vi "SerializeBuildHeader.vi"(8 "error in (no error)":errorcluster, 10 "PlaceholderData?":bool[](array[boolean]), 11 "All class layers":T1[](array[typedef])) -> (0 "error out":errorcluster, 2 "Version header":variant, 3 "Class header":variant)   [LabVIEW 2020, in "BlueSerialization.lvlib" / "BlueSerializer.lvclass"]
uses:
  BlueSerializer.lvclass
  Support/GetSerializableDataClusterClass.ctl
  Support/SerializableDataGetDataAction.ctl
  ClassNameAndVersion.ctl
  <vilib>/Utility/EditLVLibs/LibVersion.ctl
  <vilib>/Utility/error.llb/Error Cluster From Error Code.vi
  <vilib>/ErrorRing/Error Ring.xnode
  <vilib>/Utility/EditLVLibs/Edit LVLibs.lvlib
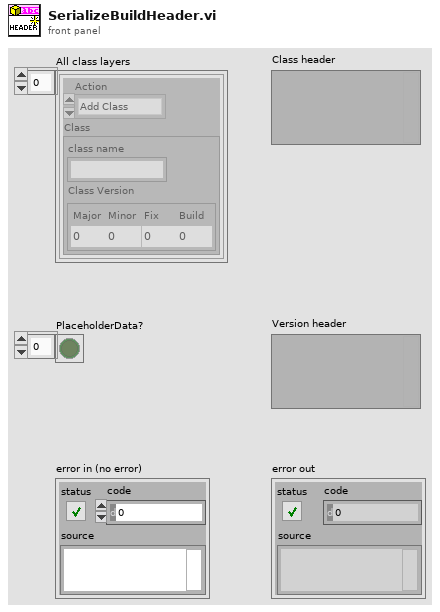
[diagram p1: front panel]
types:
  T1 = typedef "BlueSerialization.lvlib/BlueSerializer.lvclass/GetSerializableDataClusterClass.ctl" = cluster{"Action":T2, "Class":T3}
  T2 = typedef "BlueSerialization.lvlib/BlueSerializer.lvclass/SerializableDataGetDataAction.ctl" = enum16{"Add Class", "Drop Class"}
  T3 = typedef "BlueSerialization.lvlib/BlueSerializer.lvclass/ClassNameAndVersion.ctl" = cluster{"class name":string, "Class Version":T4}
  T4 = typedef "Edit LVLibs.lvlib/LibVersion.ctl" = cluster{"Major":u16, "Minor":u16, "Fix":u16, "Build":u16}
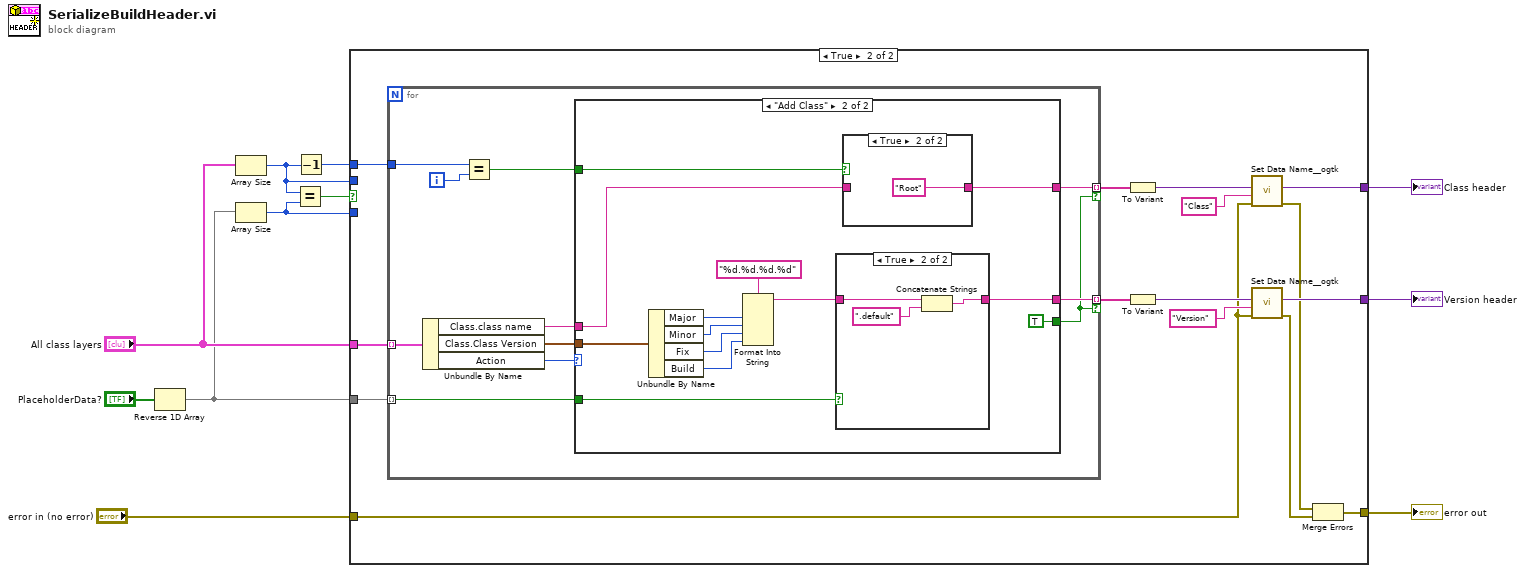
[diagram p0: block diagram]
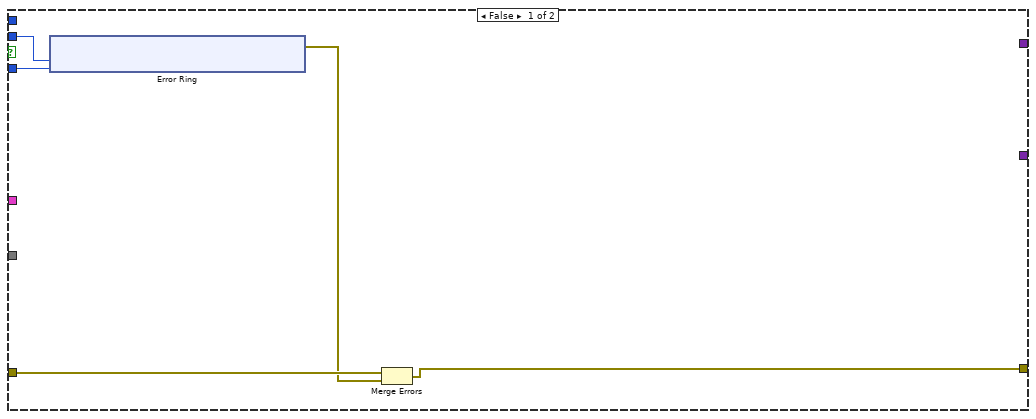
[diagram p2: hidden frame]
diagram:
  n1 = Reverse 1D Array(array="PlaceholderData?") -> (reversed array=w1:bool[])
  n2 = Array Size(array="All class layers") -> (size(s)=w3:i32)
  n3 = Array Size(array=w1) -> (size(s)=w4:i32)
  n4 = Equal?(x=w3, y=w4) -> (x = y?=w5:bool)
  n5 = Decrement(x=w3) -> (x-1=w8:i32)
  n6 = case shown="True" w5 {
    tunnel: [_ w34] -> w11
    tunnel: [_ w33] -> w10
    tunnel: "All class layers" -> [_ w32]
    tunnel: w8 -> [_ w30]
    tunnel: "error in (no error)" -> [w14 w29]
    tunnel: [w12 w27] -> w6
    tunnel: w1 -> [_ w25]
    tunnel: w4 -> [w16 _]
    tunnel: w3 -> [w15 _]
    frame False {
      n7 = xnode "Error Ring"("parameter 0"=w15, "parameter 1"=w16) -> ("error out"=w13:errorcluster)
      n8 = Merge Errors(w14, w13) -> (w12:errorcluster)
    }
    frame True {
      n9 = for {
        tunnel: w32 -> [w50] mode=indexing
        tunnel: [w48] -> w39 mode=indexing if=w44
        tunnel: [w45] -> w31 mode=indexing if=w44
        tunnel: w25 -> [w43] mode=indexing
        tunnel: w30 -> [w41]
        i -> [w42]
        n10 = Unbundle By Name(w50) -> ("Class.class name"=w46:string, "Class.Class Version"=w49:T4, "Action"=w47:T2)
        n11 = Equal?(x=w41, y=w42) -> (x = y?=w40:bool)
        n12 = case shown="\"Add Class\"" w47 {
          tunnel: w49 -> [_ w58]
          tunnel: [_ w51] -> w48
          tunnel: w46 -> [_ w55]
          tunnel: [_ w54] -> w45
          tunnel: [_ TRUE] -> w44
          tunnel: w43 -> [_ w53]
          tunnel: w40 -> [_ w56]
          frame "Drop Class" {
          }
          frame "Add Class" {
            n13 = Unbundle By Name(w58) -> ("Major"=w62:u16, "Minor"=w61:u16, "Fix"=w60:u16, "Build"=w59:u16)
            n14 = Format Into String(format string="%d.%d.%d.%d", w62, w61, w60, w59) -> (resulting string=w52:string)  [unwired: 2 in, 1 out]
            n15 = case shown="True" w53 {
              tunnel: w52 -> [w64 w67]
              tunnel: [w64 w65] -> w51
              frame False {
              }
              frame True {
                n16 = Concatenate Strings(w67, ".default" ("string")) -> (w65:string)
              }
            }
            n17 = case shown="True" w56 {
              tunnel: w55 -> [w68 _]
              tunnel: [w68 "Root" ("new element/subarray")] -> w54
              frame False {
              }
              frame True {
              }
            }
          }
        }
      }
      n18 = To Variant(anything=w31) -> (Variant=w38:variant)
      n19 = To Variant(anything=w39) -> (Variant=w35:variant)
      n20 = call <userlib>:"Set Data Name__ogtk.vi"("error in (no error)"=w29, "Data Name"="Class", "Data"=w38) -> ("error out"=w26:errorcluster, "Renamed Data"=w34:variant)  [unwired: 7 in]
      n21 = call <userlib>:"Set Data Name__ogtk.vi"("error in (no error)"=w29, "Data Name"="Version", "Data"=w35) -> ("error out"=w28:errorcluster, "Renamed Data"=w33:variant)  [unwired: 7 in]
      n22 = Merge Errors(w26, w28) -> (w27:errorcluster)
    }
  }
  "Class header" <- w11
  "Version header" <- w10
  "error out" <- w6
